vi "Save Config User Event.vi"(7 "Save Config Ref":refnum<vi>, 10 "Graph Settings":T1, 11 "Register (F)":bool) -> (3 "Save Config Event Ref":refnum<user-event>)   [LabVIEW 2019]
uses:
  Type Defs and Controls/Graph Settings Type Def.ctl
  Type Defs and Controls/Save Config Event Type Def.ctl
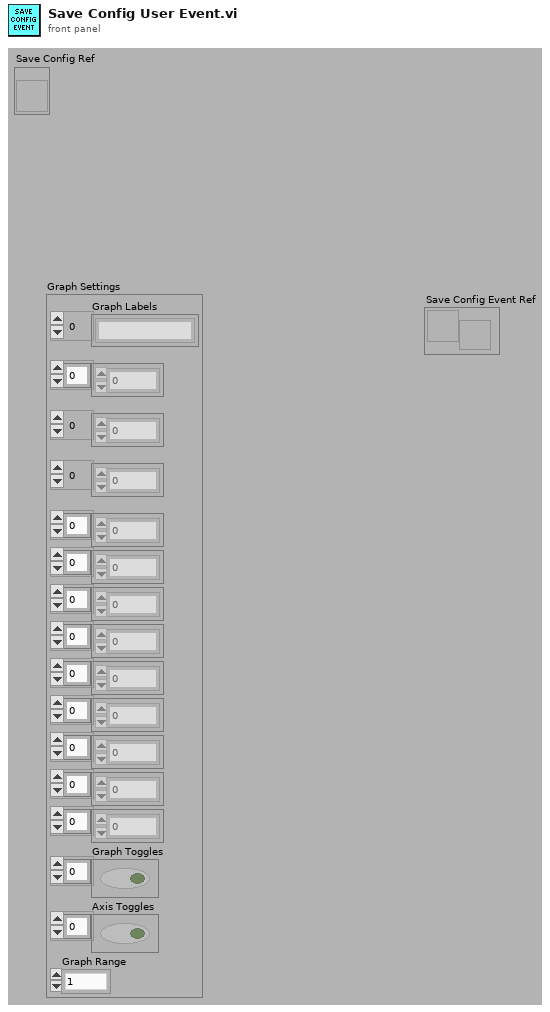
[diagram p1: front panel]
types:
  T1 = typedef "Graph Settings Type Def.ctl" = cluster{"Graph Labels":string[], u8[], i16[], u32[], u8[], u8[], u8[], u32[], u8[], u8[], u8[], dbl[], dbl[], "Graph Toggles":bool[], "Axis Toggles":bool[], "Graph Range":enum16{"1", "2", "3", "4", "5", "10", "15", "30", "60"}}
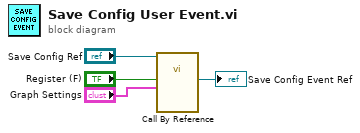
[diagram p0: block diagram]
diagram:
  n1 = call-by-ref "?"(reference="Save Config Ref", "Graph Settings"="Graph Settings", "Register (F)"="Register (F)") -> ("Save Config Event Ref"=→"Save Config Event Ref":refnum<user-event>)  [unwired: 10 in, 2 out]
